vi "test6.vi"() -> ()   [LabVIEW 2020]
panel:
  out "x+y":dbl
  in  "Stop":bool
  out "Numeric":dbl
  out "theta":dbl
  out "r":dbl
  in  "y":dbl
  in  "x":dbl
  out "XY Graph":cluster{dbl[], dbl[]}(graph)
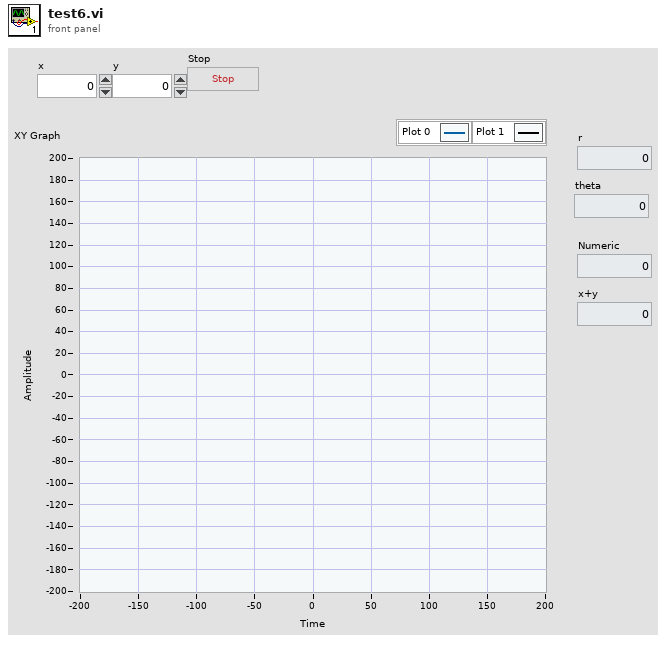
[diagram p1: front panel]
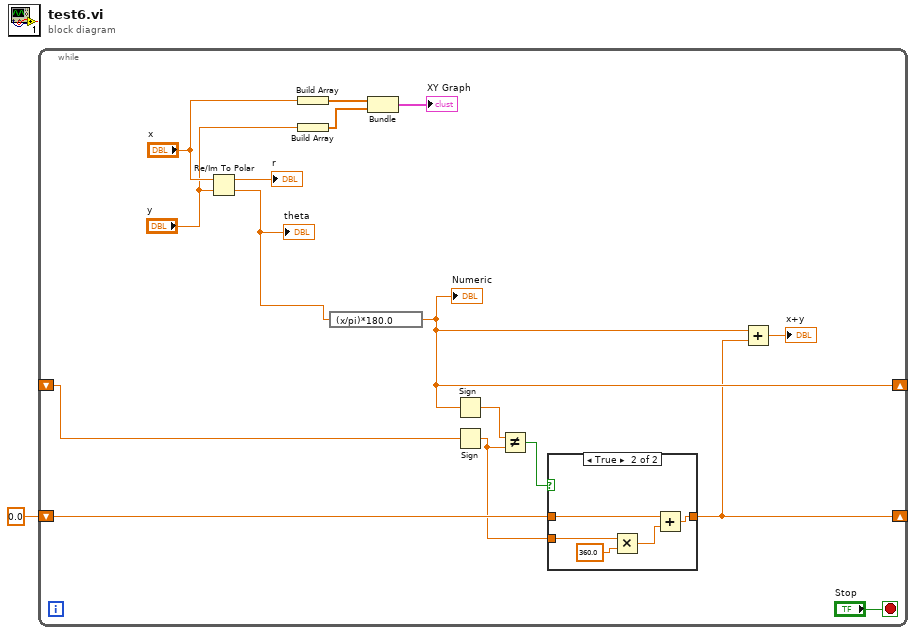
[diagram p0: block diagram]
diagram:
  n1 = while {
    shift-right: [w4] -> _
    shift-left: _ -> [w9]
    shift-right: [w3] -> _
    shift-left: 0.0 -> [w6]
    stop <- "Stop" stop-if-true
    n2 = Re/Im To Polar(2:"y", 3:"x") -> (0:w10:dbl, 1:→"r":dbl)
    "theta" <- w10
    n3 = Build Array("x") -> (w15:dbl[])
    n4 = Build Array("y") -> (w14:dbl[])
    n5 = expression code="(x/pi)*180.0"(w10) -> (w4:dbl)
    "Numeric" <- w4
    n6 = Bundle(w15, w14) -> (→"XY Graph":cluster{dbl[], dbl[]})  [unwired: 1 in]
    n7 = Sign(1:w4) -> (0:w8:dbl)
    n8 = Sign(1:w9) -> (0:w5:dbl)
    n9 = Not Equal?(x=w8, y=w5) -> (x != y?=w7:bool)
    n10 = case shown="True" w7 {
      tunnel: w6 -> [w18 w21]
      tunnel: [w18 w19] -> w3
      tunnel: w5 -> [_ w23]
      frame False {
      }
      frame True {
        n11 = Multiply(x=w23, y=360.0) -> (x*y=w20:dbl)
        n12 = Add(x=w21, y=w20) -> (x+y=w19:dbl)
      }
    }
    n13 = Add(x=w4, y=w3) -> (x+y=→"x+y":dbl)
  }
